vi "Prefilter_LP.vi"(10 "high cutoff freq [Hz]":dbl=0.45, 11 "Array":waveform(dbl)[](array[waveform])) -> (3 "Array 2":waveform(dbl)[](array[waveform]))   [LabVIEW 2016]
uses:
  <vilib>/addons/Digital Filter Design/Process.llb/DFD Filtering (Wfm NChan).vi
  <vilib>/addons/Digital Filter Design/NI_DigFilterLicensed.lvlib
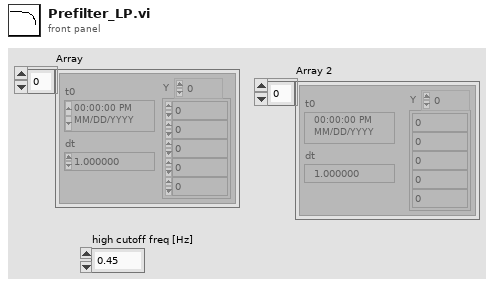
[diagram p1: front panel]
types:
  T1 = enum16{"Lowpass", "Highpass", "Bandpass", "Bandstop"}
  T2 = typedef "NI_DigFilterLicensed.lvlib/DFD Filter Obj.ctl" = cluster{"mSRate_Fs":dbl, "mSRate_Version":string, "mSRate_Comments":string, "mSRate_OrgCoef":T3, "mSRate_CurCoef":T3, "mSRate_Quantized?":bool, "mSRate_QCoef":T3, "mSRate_QSettings":T5[], "mSRate_Order":i32, "mSRate_Scaling":cluster{"mSRate_ScaleByPowerOf2?":bool, "mSRate_ScaleType":T7}}
  T3 = typedef "NI_DigFilterLicensed.lvlib/DFD Filter Coef.ctl" = cluster{"type":T4, "gain":dbl, "coef a (k)":dbl[], "coef b (v)":dbl[]}
  T4 = typedef "NI_DigFilterLicensed.lvlib/DFD Filter Structure Type Selector.ctl" = enum16{"Undefined", "FIR Direct Form", "FIR Direct Form Transposed", "FIR Symmetric", "FIR Antisymmetric", "IIR Direct Form I", "IIR Direct Form I Transposed", "IIR Direct Form II", "IIR Direct Form II Transposed", "IIR Cascaded Second Order Sections Form I", "IIR Cascaded Second Order Sections Form I Transposed", "IIR Cascaded Second Order Sections Form II", "IIR Cascaded Second Order Sections Form II Transposed", "Lattice Allpass (basic sections)", "Lattice Allpass (one multiplier sections)", "Lattice Allpass (normalized sections)", "Lattice AR (basic sections)", "Lattice AR (one multiplier sections)", "Lattice AR (normalized sections)", "Lattice MA (minimum phase)", "Lattice MA (maximum phase)", "Lattice ARMA (basic sections)", "Lattice ARMA (one multiplier sections)", "Lattice ARMA (normalized sections)"}
  T5 = typedef "NI_DigFilterLicensed.lvlib/dfd_Internal Quantization Settings.ctl" = cluster{"source":T6, "wl":i16, "iwl":i16, "overflow mode":enum16{"Saturation", "Wrap"}, "rounding mode":enum16{"Nearest", "Truncation"}, "signed?":bool}
  T6 = typedef "NI_DigFilterLicensed.lvlib/dfd_Internal Quantization Srcs.ctl" = u16
  T7 = typedef "NI_DigFilterLicensed.lvlib/DFD Coef Norm Type.ctl" = enum16{"No Norm", "Time Domain 1-Norm", "Time Domain 2-Norm", "Time Domain Inf-Norm"}
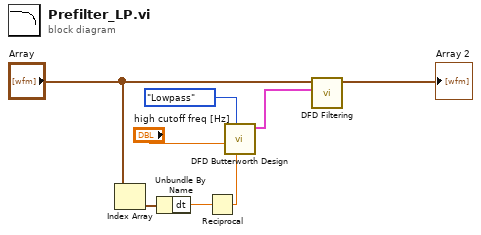
[diagram p0: block diagram]
diagram:
  n1 = Index Array(array="Array") -> (element=w7:waveform(dbl))  [unwired: 1 in]
  n2 = Unbundle By Name(w7) -> ("dt"=w8:dbl)
  n3 = Reciprocal(x=w8) -> (1/x=w4:dbl)
  n4 = call <vilib>:"DFD Butterworth Design.vi"("fs [Hz]"=w4, "filter type"=T1."Lowpass", "low cutoff freq [Hz]"="high cutoff freq [Hz]") -> ("filter out"=w3:T2)  [unwired: 7 in, 1 out]
  n5 = call-poly <vilib>:"DFD Filtering.vi"("filter"=w3, "signal in"="Array") -> ("signal out"=→"Array 2":waveform(dbl)[])  [unwired: 8 in, 1 out]
